vi "Abort Message Queue.vi"(10 "error to report":errorcluster) -> (3 "channel":T1)   [LabVIEW 2020, in "Message Queue.lvlib"]
doc: "This VI stops the message queue, raising an abort signal for all readers and writers of the channel."
uses:
  Message Queue.lvlib
  <extravilib>/ChannelInstances/Messenger-t'Message Queue.lvlib-Message Cluster.ctl'/))Channel.ctl
  Message Cluster.ctl
  <extravilib>/ChannelInstances/Messenger-t'Message Queue.lvlib-Message Cluster.ctl'/Endpoint.vi
  <extravilib>/ChannelInstances/Messenger-t'Message Queue.lvlib-Message Cluster.ctl'.lvlib
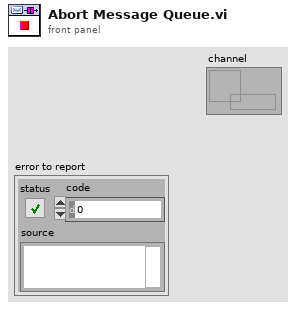
[diagram p1: front panel]
types:
  T1 = typedef "Messenger-t'Message Queue.lvlib-Message Cluster.ctl'.lvlib/))Channel.ctl" = refnum<queue>
  T2 = typedef "Message Queue.lvlib/Message Cluster.ctl" = cluster{"Message":string, "Message Data":variant}
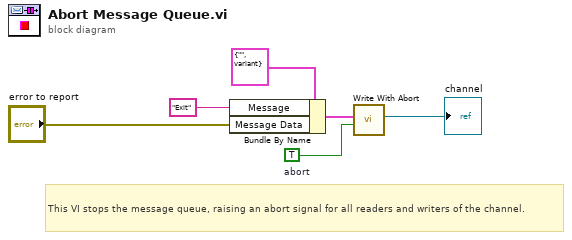
[diagram p0: block diagram]
diagram:
  w1 = TRUE  # abort
  # "This VI stops the message queue, raising an abort signal for all readers and writers of the channel."
  n1 = Bundle By Name(cluster=T2 {"Message"="", "Message Data"=variant} ("Message Cluster"), "Message"="Exit", "Message Data"="error to report") -> (w6:T2)
  n2 = call <extravilib>:"Write With Abort.vi"("abort (F)"=w1, "element"=w6) -> ("channel"=→"channel":T1)  [unwired: 6 in, 3 out]
